vi "ReverseDirection.vi"(0 "reference":refnum<class "AbstractEdge.lvclass">, 5 "error in (no error)":errorcluster) -> (14 "reference out":refnum<class "AbstractEdge.lvclass">, 19 "error out":errorcluster)   [LabVIEW 2016, in "AbstractEdge.lvclass"]
uses:
  <resource>/Framework/Providers/Open_GDS/UML/AbstractEdge_class/AbstractEdge.lvclass
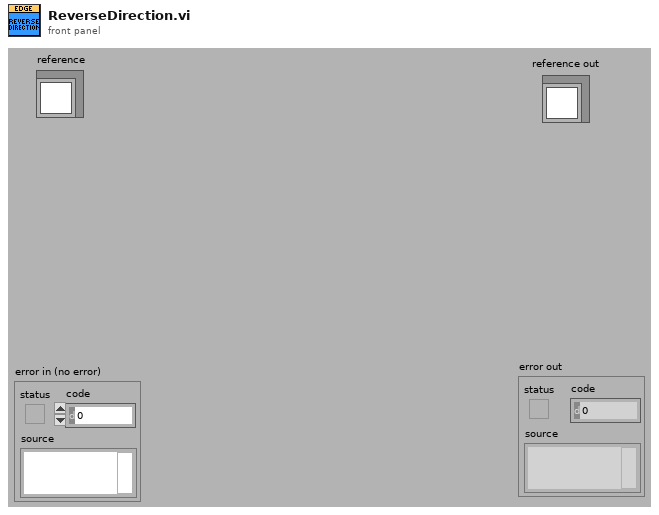
[diagram p1: front panel]
types:
  T1 = typedef "AbstractEdge.lvclass/ObjectAttributes.ctl" = cluster{"start":refnum<class "AbstractNode.lvclass">, "end":refnum<class "AbstractNode.lvclass">}
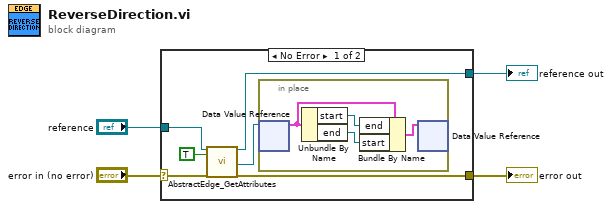
[diagram p0: block diagram]
diagram:
  n1 = case shown="No Error" "error in (no error)" {
    selector: "error in (no error)" -> [w7 w15]
    tunnel: "reference" -> [w10 w16]
    tunnel: [w9 w15] -> w3
    tunnel: [w8 w16] -> w2
    frame No Error {
      n2 = call <resource>:"AbstractEdge_GetAttributes.vi"("reference in"=w10, "OnlyGetDvrReference(False)"=TRUE, "error in (no error)"=w7) -> ("reference out"=w8:refnum<class "AbstractEdge.lvclass">, "DataRef"=w5:refnum<data-value>, "error out"=w9:errorcluster)  [unwired: 13 in, 1 out]
      n3 = in-place {
        n4 = in-place-dvr #1(w5) -> (w14:T1)  [unwired: 1 out]
        n5 = Unbundle By Name(w14) -> ("start"=w13:refnum<class "AbstractNode.lvclass">, "end"=w12:refnum<class "AbstractNode.lvclass">)
        n6 = Bundle By Name(cluster=w14, "end"=w13, "start"=w12) -> (w11:T1)
        n7 = in-place-dvr #1(w11) -> ()  [unwired: 2 out]
      }
    }
    frame Error {
    }
  }
  "reference out" <- w2
  "error out" <- w3
